vi "Throw.vi"(0 "Throw?":bool, 9 "MotorControlDevRef":T1={"DeviceStatus"={"status"=FALSE, "code"=0, "source"=""}, "Type"=enum."PWM", "PWM"={"Digital Module"=enum."Digital Module 1", "PWM Channel"=enum."Invalid", "DeadBand"={"Name"="", "maxPositivePwm"=0, "minPositivePwm"=0, "centerPwm"=0, "maxNegativePwm"=0, "minNegativePwm"=0, "angularRange"=0}}, "CAN"={"Device Number"=0, "Control Mode"=enum."Percent VBus", "Semaphore"=refnum, "Max Vout"=12.0}, "Invert"=FALSE, "TransformRef"=refnum, "InvTransformRef"=refnum}, 11 "Engage latch":bool) -> ()   [LabVIEW 2013]
uses:
  Events.vi
  <vilib>/Rock Robotics/WPI/PWM/WPI_PWMTransform_ConPane.ctl
  <vilib>/Rock Robotics/SystemInterfaces/Typedef/FPGA_TypedefDigitalModule.ctl
  <vilib>/Rock Robotics/SystemInterfaces/DIO/FPGA_DIOPWMChannel.ctl
  <vilib>/Rock Robotics/WPI/PWM/WPI_PWMDeadband.ctl
  <vilib>/Rock Robotics/WPI/CAN/Jaguar/SubVIs/WPI_CANJaguar_ControlMode.ctl
  <vilib>/Rock Robotics/WPI/MotorControl/WPI_MotorControlDeviceRef.ctl
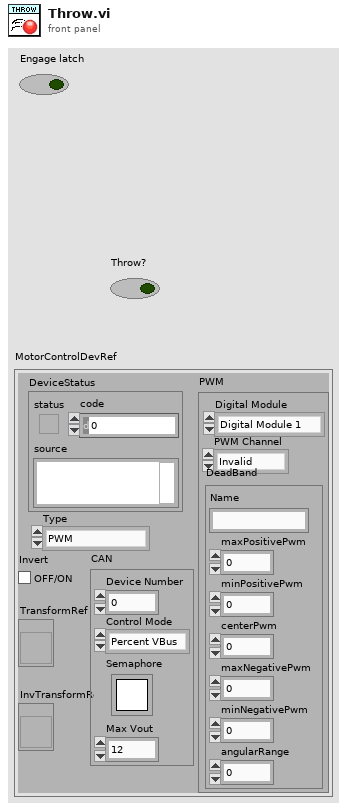
[diagram p1: front panel]
types:
  T1 = typedef "WPI_MotorControlDeviceRef.ctl" = cluster{"DeviceStatus":errorcluster, "Type":enum16{"PWM", "CAN"}, "PWM":cluster{"Digital Module":T2, "PWM Channel":T3, "DeadBand":T4}, "CAN":cluster{"Device Number":u8, "Control Mode":T5, "Semaphore":T6, "Max Vout":dbl}, "Invert":bool, "TransformRef":T7, "InvTransformRef":T7}
  T2 = typedef "FPGA_TypedefDigitalModule.ctl" = enum16{"Digital Module 1", "Digital Module 2"}
  T3 = typedef "FPGA_DIOPWMChannel.ctl" = enum8{"PWM 1", "PWM 2", "PWM 3", "PWM 4", "PWM 5", "PWM 6", "PWM 7", "PWM 8", "PWM 9", "PWM 10", "Invalid"}
  T4 = typedef "WPI_PWMDeadband.ctl" = cluster{"Name":string, "maxPositivePwm":i32, "minPositivePwm":i32, "centerPwm":i32, "maxNegativePwm":i32, "minNegativePwm":i32, "angularRange":u16}
  T5 = typedef "WPI_CANJaguar_ControlMode.ctl" = enum8{"Percent VBus", "Current", "Speed", "Position", "Voltage"}
  T6 = typedef "Semaphore RefNum" = refnum<k1>
  T7 = typedef "WPI_PWMTransform_ConPane.ctl" = refnum<vi>
  T8 = enum16{"Fire (Release latch)", "Wait for fire", "Engage latch", "Do Nothing"}
  T9 = cluster{"axis 1":dbl, "axis 2":dbl, "axis 3":dbl, "axis 4":dbl, "axis 5":dbl, "Change Power":dbl}
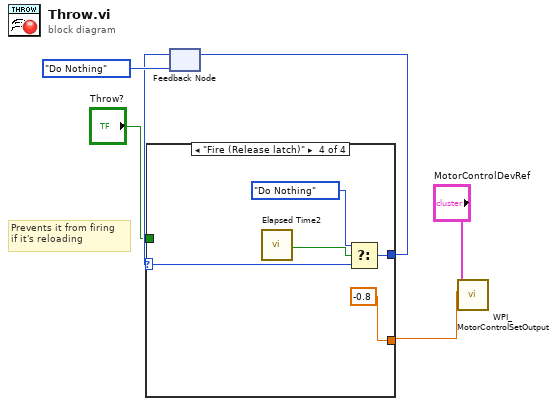
[diagram p0: block diagram]
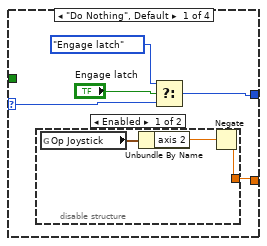
[diagram p2: hidden frame]
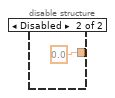
[diagram p3: hidden frame]
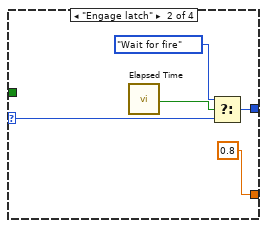
[diagram p4: hidden frame]
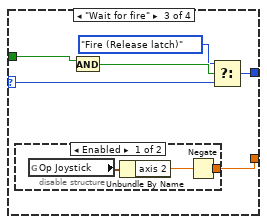
[diagram p5: hidden frame]
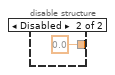
[diagram p6: hidden frame]
diagram:
  # "Prevents it from firing \nif it's reloading"
  n1 = feedback #1(T8."Do Nothing") -> (w5:T8)
  n2 = case shown="\"Fire (Release latch)\"" w5 {
    selector: w5 -> [w10 w19 w24 w31]
    tunnel: [w7 w18 w22 w32] -> w4
    tunnel: [w8 0.8 w21 -0.8] -> w2
    tunnel: "Throw?" -> [_ _ w26 _]
    frame "Do Nothing", Default {
      n3 = disable-structure shown="Enabled" {
        disable-tunnel: [w12 0.0] -> w8
        frame Enabled {
          n4 = global read "Events.vi" "Op Joystick"() -> (w14:T9)
          n5 = Unbundle By Name(w14) -> ("axis 2"=w13:dbl)
          n6 = Negate(x=w13) -> (-x=w12:dbl)
        }
        frame Disabled {
        }
      }
      n7 = Select(t=T8."Engage latch", s="Engage latch", f=w10) -> (s? t:f=w7:T8)
    }
    frame "Engage latch" {
      n8 = call "Elapsed Time"() -> ("Time has Elapsed"=w16:bool)  [unwired: 12 in, 7 out]
      n9 = Select(t=T8."Wait for fire", s=w16, f=w19) -> (s? t:f=w18:T8)
    }
    frame "Wait for fire" {
      n10 = disable-structure shown="Enabled" {
        disable-tunnel: [w27 0.0] -> w21
        frame Enabled {
          n11 = global read "Events.vi" "Op Joystick"() -> (w29:T9)
          n12 = Unbundle By Name(w29) -> ("axis 2"=w28:dbl)
          n13 = Negate(x=w28) -> (-x=w27:dbl)
        }
        frame Disabled {
        }
      }
      n14 = And(x=w26) -> (x .and. y?=w25:bool)  [unwired: 1 in]
      n15 = Select(t=T8."Fire (Release latch)", s=w25, f=w24) -> (s? t:f=w22:T8)
    }
    frame "Fire (Release latch)" {
      n16 = call "Elapsed Time2"() -> ("Time has Elapsed"=w33:bool)  [unwired: 12 in, 7 out]
      n17 = Select(t=T8."Do Nothing", s=w33, f=w31) -> (s? t:f=w32:T8)
    }
  }
  n18 = feedback-in #1(w4) -> ()
  n19 = call <vilib>:"WPI_MotorControlSetOutput.vi"("Output"=w2, "MotorControlDevRef"="MotorControlDevRef") -> ()  [unwired: 7 in, 3 out]
